vi "loadDataIntoScript_multi.vi"(8 "error in (no error)":errorcluster, 9 "Path":path=path "C:/Users/Administrator/Desktop/Crete/Lua/Sweeping/lvScript.tsp", 10 "data":dbl[][][](array[numeric]), 11 "K2602 in":refnum<class "K2602.lvclass">) -> (0 "error out":errorcluster, 2 "script":string, 3 "K2602 out":refnum<class "K2602.lvclass">)   [LabVIEW 2011, in "Hardware.lvlib" / "Channels.lvlib" / "K2602.lvclass"]
uses:
  K2602.lvclass
  K2602.lvclass/K2602.ctl
  AnalogOutput.lvclass
panel:
  out "channelConfig":string
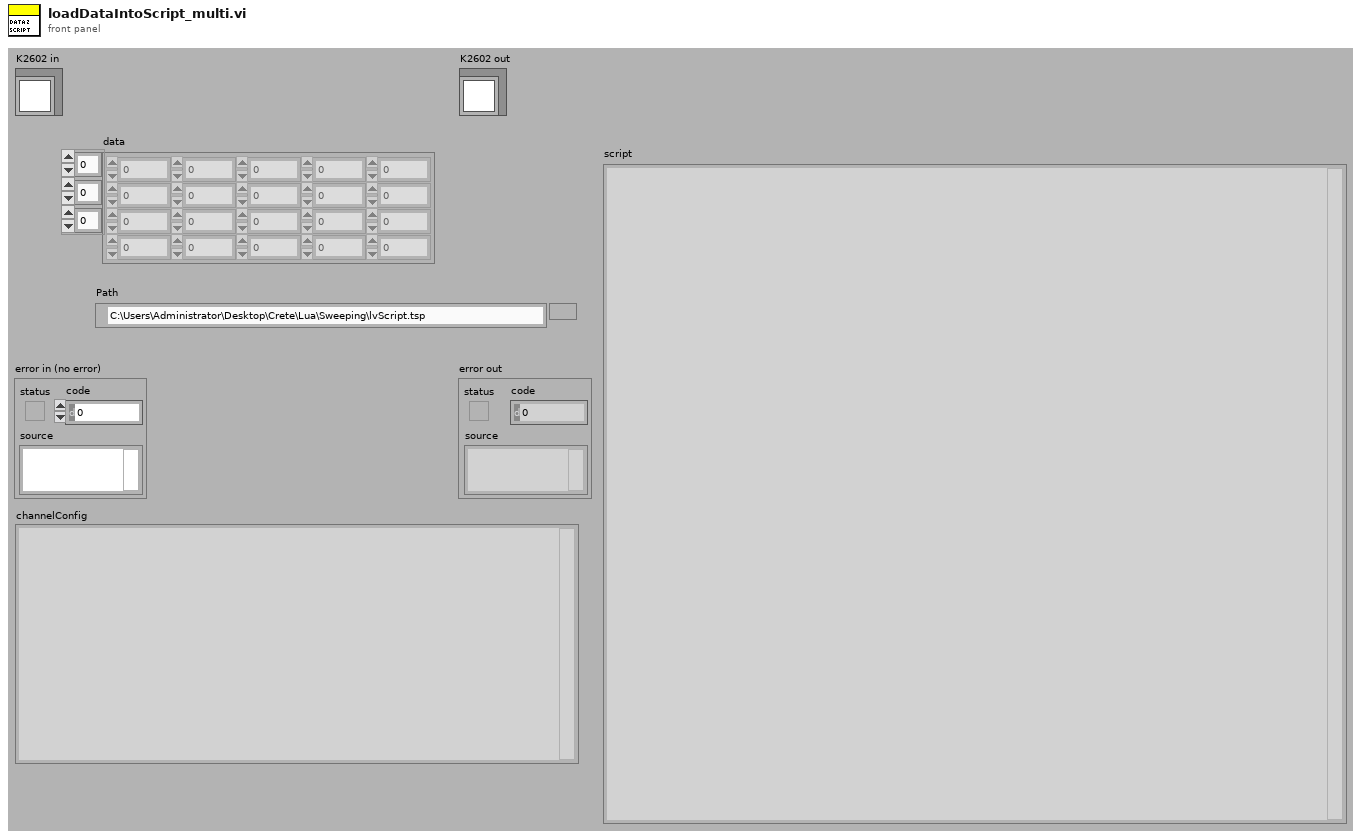
[diagram p1: front panel]
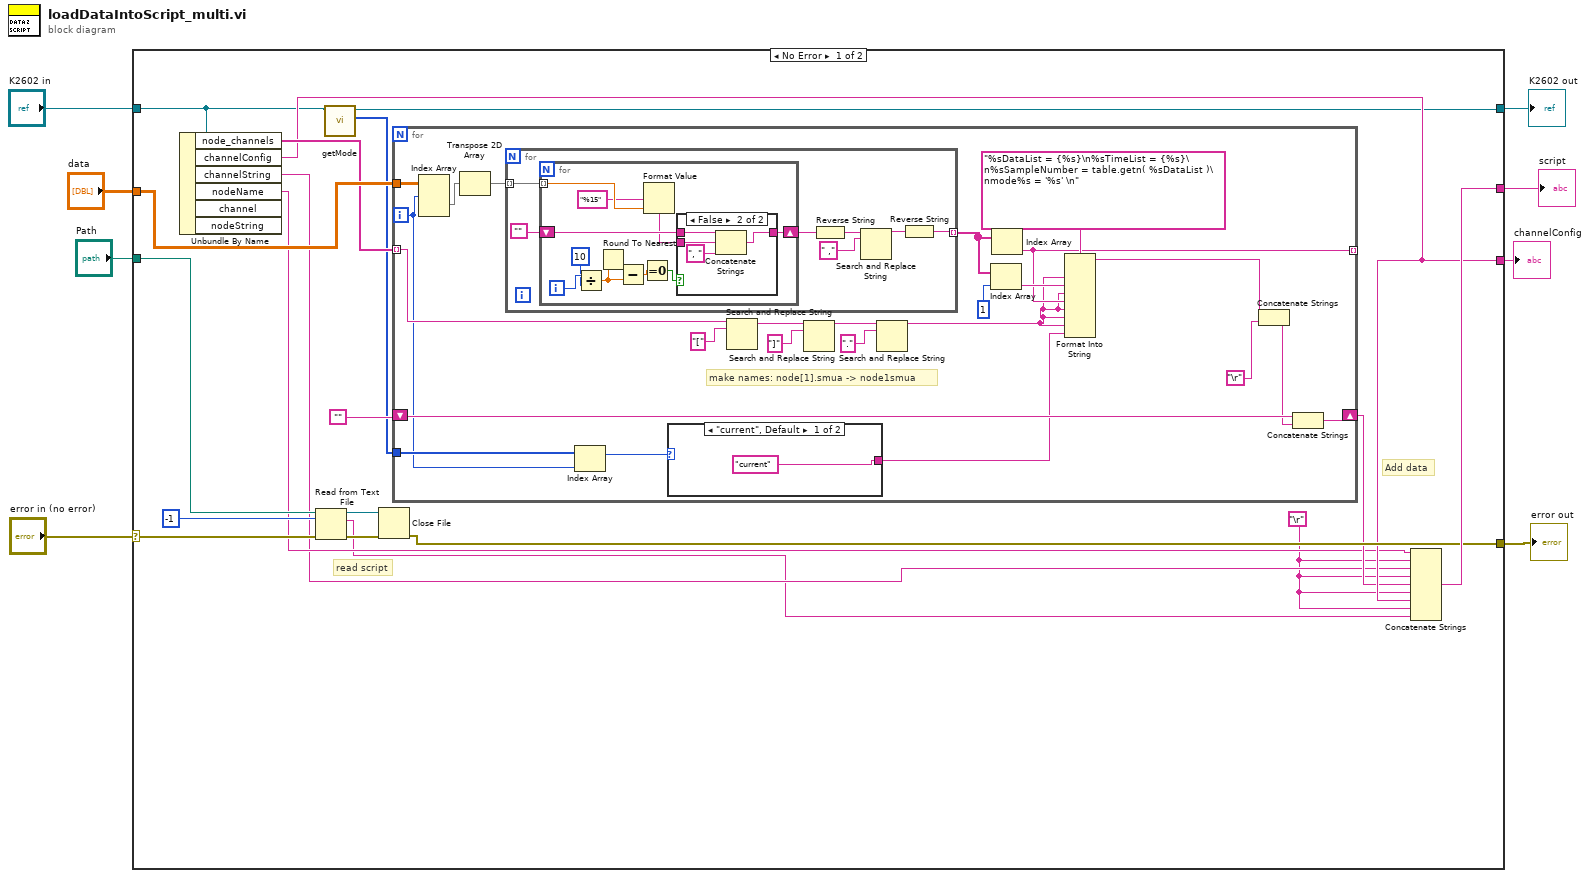
[diagram p0: block diagram]
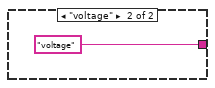
[diagram p2: hidden frame]
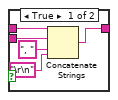
[diagram p3: hidden frame]
diagram:
  n1 = case shown="No Error" "error in (no error)" {
    selector: "error in (no error)" -> [w25 w82]
    tunnel: [w18 w82] -> w7
    tunnel: [w9 w81] -> w5
    tunnel: "K2602 in" -> [w11 w81]
    tunnel: "data" -> [w24 _]
    tunnel: "Path" -> [w27 _]
    tunnel: [w23 _] -> w2
    tunnel: [w17 _] -> w1
    frame No Error {
      w13 = "\r"
      # "Add data"
      # "read script"
      n2 = Unbundle By Name(w11) -> ("node_channels"=w21:string[], "channelConfig"=w17:string, "channelString"=w14:string, "nodeName"=w15:string)  [unwired: 2 out]
      n3 = Read from Text File(file (use dialog)=w27, count=-1, error in=w25) -> (refnum out=w20:refnum<file>, text=w12:string, error out=w19:errorcluster)  [unwired: 1 in, 1 out]
      n4 = call "getMode.vi"("AnalogOutput in"=w11) -> ("mode"=w10:enum16{"current", "voltage"}[], "AnalogOutput out"=w9:refnum<class "K2602.lvclass">)  [unwired: 8 in, 1 out]
      n5 = Close File(refnum=w20, error in=w19) -> (error out=w18:errorcluster)  [unwired: 1 out]
      n6 = for {
        tunnel: w24 -> [w41]
        tunnel: [w44] -> _ mode=indexing
        shift-right: [w49] -> w16
        shift-left: "" -> [w48]
        tunnel: w21 -> [w38] mode=indexing
        tunnel: w10 -> [w31]
        i -> [w30]
        # "make names: node[1].smua -> node1smua"
        n7 = Index Array(array=w41, index (dim 0)=w30) -> (element=w40:dbl[][])  [unwired: 2 in]
        n8 = Transpose 2D Array(2D array=w40) -> (transposed array=w43:dbl[][])
        n9 = for {
          tunnel: w43 -> [w60] mode=indexing
          tunnel: [w54] -> w50 mode=indexing
          n10 = for {
            tunnel: w60 -> [w71] mode=indexing
            shift-right: [w67] -> w58
            shift-left: "" -> [w69]
            i -> [w62]
            n11 = Divide(x=w62, y=10) -> (x/y=w64:dbl)
            n12 = Round To Nearest(number=w64) -> (nearest integer value=w65:dbl)
            n13 = Subtract(x=w65, y=w64) -> (x-y=w66:dbl)
            n14 = Equal To 0?(x=w66) -> (x = 0?=w63:bool)
            n15 = Format Value(format string="%15", value (0)=w71) -> (output string=w68:string)  [unwired: 1 in]
            n16 = case shown="False" w63 {
              tunnel: w69 -> [w76 w80]
              tunnel: w68 -> [w75 w79]
              tunnel: [w73 w77] -> w67
              frame True {
                n17 = Concatenate Strings(w76, w75, ", ", "\r\n") -> (w73:string)
              }
              frame False {
                n18 = Concatenate Strings(w80, w79, ", ") -> (w77:string)
              }
            }
          }
          n19 = Reverse String(1:w58) -> (0:w57:string)
          n20 = Search and Replace String(input string=w57, search string=" ,") -> (result string=w55:string)  [unwired: 6 in, 3 out]
          n21 = Reverse String(1:w55) -> (0:w54:string)
        }
        n22 = Index Array(array=w31, index=w30) -> (element=w32:enum16{"current", "voltage"})
        n23 = case shown="\"current\", Default" w32 {
          tunnel: ["current" "voltage"] -> w28
          frame "current", Default {
          }
          frame "voltage" {
          }
        }
        n24 = Search and Replace String(input string=w38, search string="[") -> (result string=w34:string)  [unwired: 6 in, 3 out]
        n25 = Search and Replace String(input string=w34, search string="]") -> (result string=w33:string)  [unwired: 6 in, 3 out]
        n26 = Search and Replace String(input string=w33, search string=".") -> (result string=w29:string)  [unwired: 6 in, 3 out]
        n27 = Index Array(array=w50, index=1) -> (element=w47:string)
        n28 = Index Array(array=w50) -> (element=w44:string)  [unwired: 1 in]
        n29 = Format Into String(format string="%sDataList = {%s}\n%sTimeList = {%s}\n%sSampleNumber = table.getn( %sDataList )\nmode%s = '%s' \n", w29, w47, w29, w44, w29, w29, w29, w28) -> (resulting string=w45:string)  [unwired: 2 in, 1 out]
        n30 = Concatenate Strings(w45, "\r") -> (w39:string)
        n31 = Concatenate Strings(w48, w39) -> (w49:string)
      }
      n32 = Concatenate Strings(w15, w13, w14, w13, w16, w13, w17, w13, w12) -> (w23:string)
    }
    frame Error {
    }
  }
  "error out" <- w7
  "K2602 out" <- w5
  "script" <- w2
  "channelConfig" <- w1
